vi "Enable Disable Bitfile Buttons.vi"(4 "Set Master in":refnum<vi>, 5 "Remove in":refnum<vi>, 6 "Reload in":refnum<vi>, 7 "Add in":refnum<vi>, 8 "error in (no error)":errorcluster, 9 "listbox text":string[][](array[string]), 10 "Selected Values":i32[](array[numeric]), 11 "Item Ref in":T1 format="%.0x") -> (0 "error out":errorcluster, 2 "Selected Values":i32[](array[numeric]), 3 "Item Ref out":T1 format="%.0x")   [LabVIEW 2020, in "Engine Simulation Toolkit System Explorer.lvlib"]
uses:
  Engine Simulation Toolkit System Explorer.lvlib
  <vilib>/NI VeriStand/Custom Device API/Custom Device Item Ref.ctl
  Shared/Constants and GUIDs.vi
  Shared/Properties.vi
  <vilib>/NI VeriStand/Custom Device API/Get Item Property (String).vi
  Shared/Engine Simulation Toolkit Shared.lvlib
  <vilib>/NI VeriStand/Custom Device API/Custom Device API.lvlib
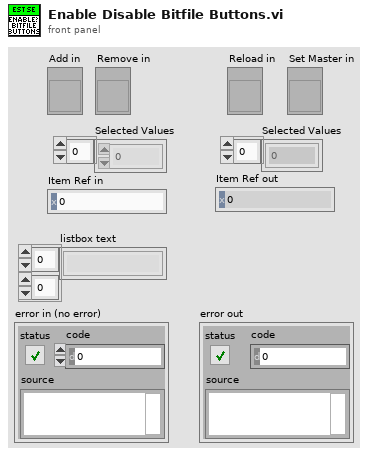
[diagram p1: front panel]
types:
  T1 = typedef "Custom Device API.lvlib/Custom Device Item Ref.ctl" = u64
  T2 = enum8{"Enabled", "Disabled", "Disabled and Grayed Out"}
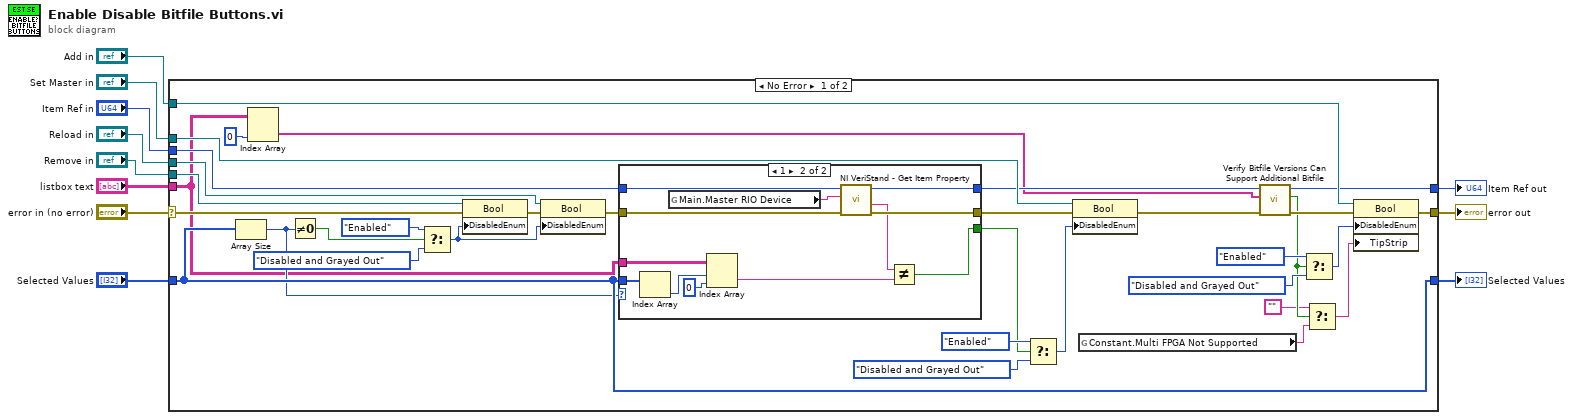
[diagram p0: block diagram]
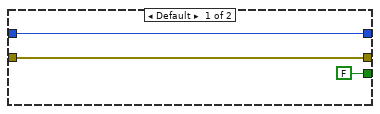
[diagram p2: hidden frame]
diagram:
  n1 = case shown="No Error" "error in (no error)" {
    selector: "error in (no error)" -> [w24 w63]
    tunnel: "Reload in" -> [w40 _]
    tunnel: "Remove in" -> [w39 _]
    tunnel: "Selected Values" -> [w34 w62]
    tunnel: [w30 w63] -> w7
    tunnel: [w34 w62] -> w6
    tunnel: "Add in" -> [w29 _]
    tunnel: "Set Master in" -> [w35 _]
    tunnel: "listbox text" -> [w23 _]
    tunnel: "Item Ref in" -> [w31 w61]
    tunnel: [w19 w61] -> w1
    frame No Error {
      n2 = Array Size(array=w34) -> (size(s)=w32:i32)
      n3 = Index Array(array=w23, index (col)=0 ("disabled index (col)")) -> (element=w17:string[])  [unwired: 1 in]
      n4 = Not Equal To 0?(x=w32) -> (x != 0?=w41:bool)
      n5 = Select(t=T2."Enabled" ("Disabled"), s=w41, f=T2."Disabled and Grayed Out" ("Disabled")) -> (s? t:f=w45:T2)
      n6 = property on="Property Node" class="Bool"(reference=w39, error in=w24, "DisabledEnum"=w45) -> (error out=w44:errorcluster)  [unwired: 1 out]
      n7 = property on="Property Node" class="Bool"(reference=w40, error in=w44, "DisabledEnum"=w45) -> (error out=w25:errorcluster)  [unwired: 1 out]
      n8 = case shown="1" w32 {
        tunnel: w34 -> [_ w60]
        tunnel: w23 -> [_ w59]
        tunnel: [FALSE w49] -> w33
        tunnel: w25 -> [w47 w56]
        tunnel: [w47 w55] -> w26
        tunnel: w31 -> [w46 w54]
        tunnel: [w46 w53] -> w18
        frame Default {
        }
        frame 1 {
          n9 = Index Array(array=w60) -> (element=w58:i32)  [unwired: 1 in]
          n10 = global read "Properties.vi" "Main.Master RIO Device"() -> (w52:string)
          n11 = Index Array(array=w59, index (row)=w58, index (col)=0 ("disabled index (col)")) -> (element=w51:string)
          n12 = call-poly <vilib>:"NI VeriStand - Get Item Property.vi"("error in (no error)"=w56, "Property Name"=w52, "Item Ref in"=w54) -> ("error out"=w55:errorcluster, "Value"=w50:string, "Item Ref out"=w53:T1)  [unwired: 5 in, 1 out]
          n13 = Not Equal?(x=w50, y=w51) -> (x != y?=w49:bool)
        }
      }
      n14 = Select(t=T2."Enabled" ("Disabled"), s=w33, f=T2."Disabled and Grayed Out" ("Disabled")) -> (s? t:f=w36:T2)
      n15 = property on="Property Node" class="Bool"(reference=w35, error in=w26, "DisabledEnum"=w36) -> (error out=w21:errorcluster)  [unwired: 1 out]
      n16 = global read "Constants and GUIDs.vi" "Constant.Multi FPGA Not Supported"() -> (w12:string)
      n17 = call "Verify Bitfile Versions Can Support Additional Bitfile.vi"("error in (no error)"=w21, "RIO Device Addresses"=w17, "Item Ref in"=w18) -> ("error out"=w20:errorcluster, "Can Add?"=w15:bool, "Item Ref out"=w19:T1)  [unwired: 6 in]
      n18 = Select(t=T2."Enabled" ("Disabled"), s=w15, f=T2."Disabled and Grayed Out" ("Disabled")) -> (s? t:f=w16:T2)
      n19 = Select(t="", s=w15, f=w12) -> (s? t:f=w14:string)
      n20 = property on="Property Node" class="Bool"(reference=w29, error in=w20, "DisabledEnum"=w16, "TipStrip"=w14) -> (error out=w30:errorcluster)  [unwired: 1 out]
    }
    frame Error {
    }
  }
  "Selected Values" <- w6
  "error out" <- w7
  "Item Ref out" <- w1
